vi "Read Forces.vi"(8 "error in":errorcluster, 11 "ChanMngOOB_Rx in":refnum<class "ChanMngOOB_Rx.lvclass">) -> (0 "error out":errorcluster, 1 "Offset":i32, 2 "Forces":T1[](array[typedef]) {"Force Data" format="%x"}, 3 "ChanMngOOB_Rx out":refnum<class "ChanMngOOB_Rx.lvclass">)   [LabVIEW 2021, in "ChanMngOOB_Rx.lvclass"]
uses:
  ChanMngOOB_Rx.lvclass
  ChanMngOOB_Rx.lvclass/ChanMngOOB_Rx.ctl
  Typedef/Channel Fault Data.ctl
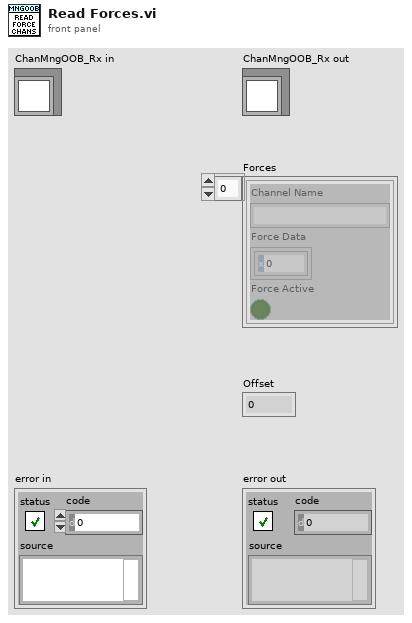
[diagram p1: front panel]
types:
  T1 = typedef "ChanMngOOB_Rx.lvclass/Channel Fault Data.ctl" = cluster{"Channel Name":string, "Force Data":u8[], "Force Active":bool}
  T2 = typedef "ChanMngOOB_Rx.lvclass/Template Payload.ctl" = cluster{"Connections":T3[], "Forces":T1[], "FIFO Pub":T4}
  T3 = typedef "ChanMngOOB_Rx.lvclass/Channel Connection Data.ctl" = cluster{"Publisher Name":string, "Subscriber Name":string, "Connection Data":u8[]}
  T4 = typedef "ChanMngOOB_Rx.lvclass/FIFO Publisher.ctl" = cluster{"Publisher Name":string, "New FIFO Instance Config":T5}
  T5 = typedef "ChannelCommon.lvlib/New FIFO Instance Configuration.ctl" = cluster{"Primary":bool, "Backpressure":bool, "Message/FIFO Override":u32}
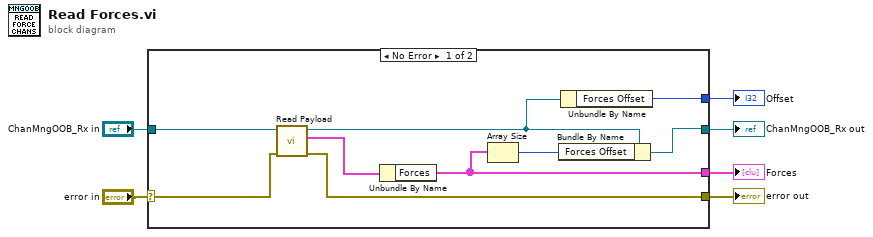
[diagram p0: block diagram]
diagram:
  n1 = case shown="No Error" "error in" {
    selector: "error in" -> [w15 w17]
    tunnel: [w13 w17] -> w6
    tunnel: [w11 w16] -> w5
    tunnel: "ChanMngOOB_Rx in" -> [w12 w16]
    tunnel: [w8 _] -> w1
    tunnel: [w9 _] -> w2
    frame No Error {
      n2 = call "Read Payload.vi"("error in"=w15, "ChanMngOOB_Rx in"=w12) -> ("error out"=w13:errorcluster, "data"=w14:T2, "ChanMngOOB_Rx out"=w10:refnum<class "ChanMngOOB_Rx.lvclass">)  [unwired: 7 in]
      n3 = Unbundle By Name(w14) -> ("Forces"=w8:T1[])
      n4 = Array Size(array=w8) -> (size(s)=w7:i32)
      n5 = Bundle By Name(cluster=w10, "Forces Offset"=w7) -> (w11:refnum<class "ChanMngOOB_Rx.lvclass">)
      n6 = Unbundle By Name(w10) -> ("Forces Offset"=w9:i32)
    }
    frame Error {
    }
  }
  "error out" <- w6
  "ChanMngOOB_Rx out" <- w5
  "Offset" <- w2
  "Forces" <- w1
